vi "Configure Temperature Measurement.vi"(8 "error in (no error)":errorcluster, 10 "Temperature Offset (-7 )":sgl=-7.0 min=-40 max=40 format="%#_6f", 11 "VISA resource name":refnum<visa-resource-name>) -> (0 "error out":errorcluster, 3 "VISA resource out":refnum<visa-resource-name>)   [LabVIEW 2011, in "Ocean Server OS4000.lvlib"]
doc: "Set Temperature offset in O.1C. Example: +-131 will subtract 13.1 from the reported temperature."
uses:
  Ocean Server OS4000.lvlib
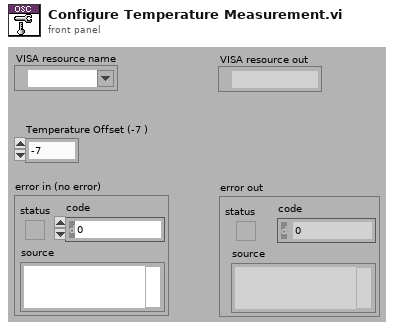
[diagram p1: front panel]
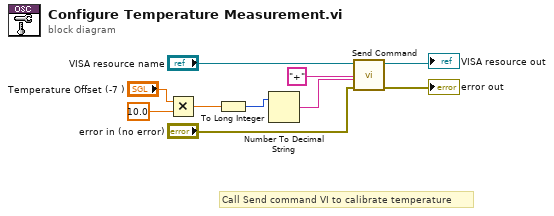
[diagram p0: block diagram]
diagram:
  # "Call Send command VI to calibrate temperature"
  n1 = Multiply(x="Temperature Offset (-7 )", y=10.0) -> (x*y=w2:dbl)
  n2 = To Long Integer(number=w2) -> (32bit integer=w1:i32)
  n3 = Number To Decimal String(number=w1) -> (decimal integer string=w8:string)  [unwired: 1 in]
  n4 = call "Send Command.vi"("error in (no error)"="error in (no error)", "Value"=w8, "Message"="+", "VISA resource name"="VISA resource name") -> ("error out"=→"error out":errorcluster, "VISA resource out"=→"VISA resource out":refnum<visa-resource-name>)  [unwired: 6 in]
